vi "Write Replace existing.vi"(8 "error in (no error)":errorcluster, 10 "Replace existing":bool, 11 "SQLite configuration in":refnum<class "SQLite configuration.lvclass">) -> (0 "error out":errorcluster, 3 "SQLite configuration out":refnum<class "SQLite configuration.lvclass">)   [LabVIEW 2014, in "SQLite configuration.lvclass"]
uses:
  SQLite configuration.lvclass
  SQLite configuration.lvclass/SQLite configuration.ctl
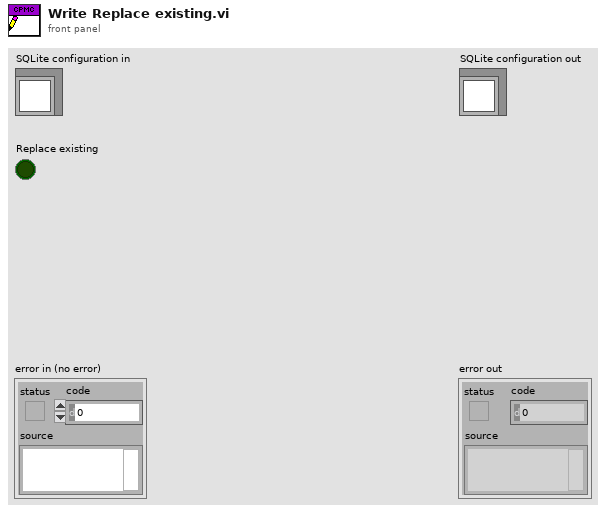
[diagram p1: front panel]
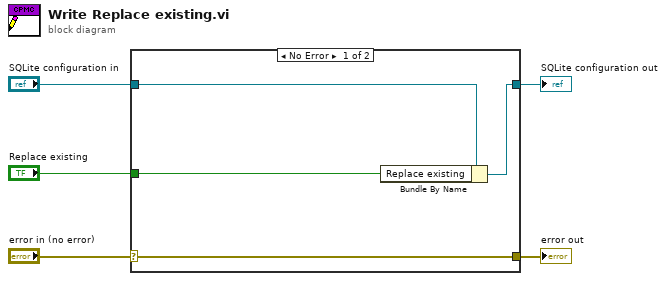
[diagram p0: block diagram]
diagram:
  n1 = case shown="No Error" "error in (no error)" {
    selector: "error in (no error)" -> [w9 w10]
    tunnel: [w9 w10] -> w4
    tunnel: [w7 w11] -> w2
    tunnel: "SQLite configuration in" -> [w8 w11]
    tunnel: "Replace existing" -> [w6 _]
    frame No Error {
      n2 = Bundle By Name(cluster=w8, "Replace existing"=w6) -> (w7:refnum<class "SQLite configuration.lvclass">)
    }
    frame Error {
    }
  }
  "error out" <- w4
  "SQLite configuration out" <- w2
